vi "Logger Global.vi"() -> ()   [LabVIEW 2018]
panel:
  out "Error Log File Count":u16
  out "Server Active?":bool
  out "Server Status":bool=TRUE
  out "Log File Count":u16
  out "Line Count":u16
  out "File Ref Out":refnum<file>
  in  "Current Queue Name":string
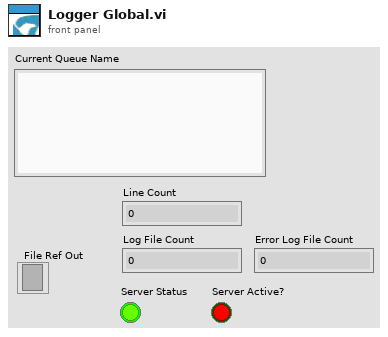
[diagram p1: front panel]
diagram:
